vi "SET_START_STOP_MEASURE.vi"(7 "LabVIEW Web Service Request":refnum<class "Web Request.lvclass">, 10 "TRIGGER":bool=TRUE, 11 "DEVICE_SN":string) -> (3 "Response":T1)   [LabVIEW 2015]
uses:
  <vilib>/wsapi/Web Request.lvclass
  Share Data/uPower_kit.ctl
panel:
  # "Use the Web Service Request input terminal to call the VIs on the Web Services palette. Do not remove it from the connector pane unless you don't need access to the palette."
  # "Each additional control wired to the connector pane will be available as an input in the URL. To include an indicator in terminal-mode output (the default setting), it must also be wired to the connector pane."
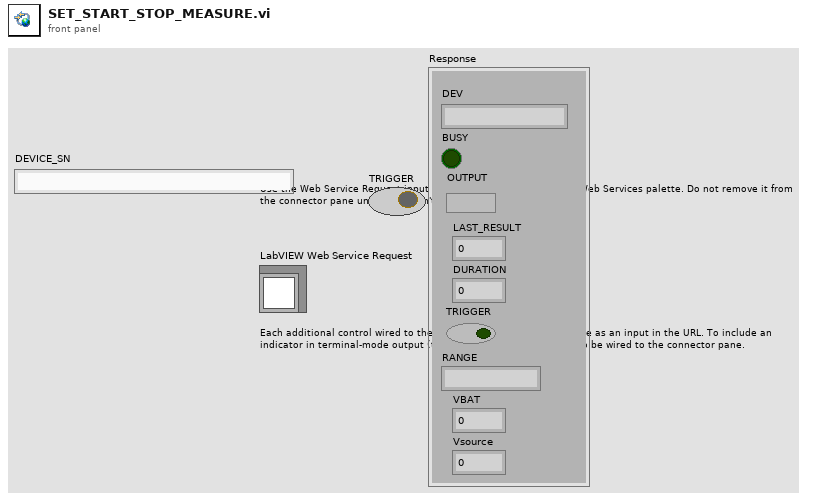
[diagram p1: front panel]
types:
  T1 = typedef "uPower_kit.ctl" = cluster{"DEV":string, "BUSY":bool, "VBAT":dbl, "OUTPUT":bool, "LAST_RESULT":dbl, "DURATION":u16, "TRIGGER":bool, "RANGE":string, "Vsource":dbl}
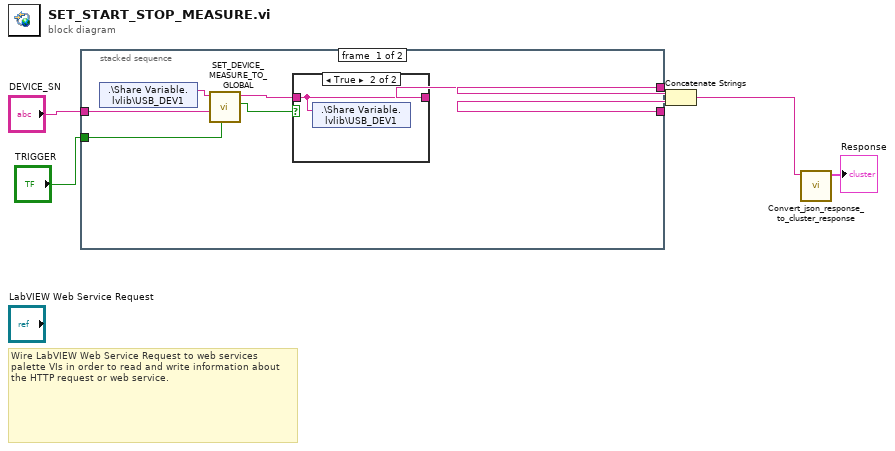
[diagram p0: block diagram]
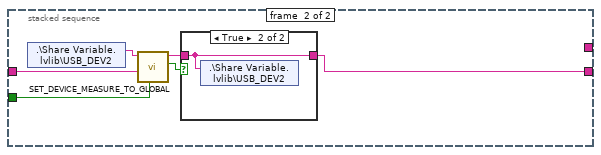
[diagram p3: hidden frame]
diagram:
  # "Wire LabVIEW Web Service Request to web services palette VIs in order to read and write information about the HTTP request or web service."
  n1 = stacked-sequence {
    tunnel: "DEVICE_SN" -> [w11 w18]
    tunnel: "TRIGGER" -> [w10 w17]
    tunnel: [w7 _] -> w4
    tunnel: [_ w14] -> w3
    frame #0 {
      n2 = shared-variable ".\\Share Variable.lvlib\\USB_DEV1"() -> (w12:string)  [unwired: 1 in, 1 out]
      n3 = call "SET_DEVICE_MEASURE_TO_GLOBAL.vi"("TRIGGER"=w10, "DEVICE in"=w11, "USB_DEV"=w12) -> ("DEVICE? 2"=w9:bool, "JSON string response 2"=w8:string)  [unwired: 7 in]
      n4 = case shown="True" w9 {
        tunnel: w8 -> [_ w13]
        tunnel: [_ w13] -> w7
        frame False {
        }
        frame True {
          n5 = shared-variable ".\\Share Variable.lvlib\\USB_DEV1"(w13) -> ()  [unwired: 1 in, 1 out]
        }
      }
    }
    frame #1 {
      n6 = shared-variable ".\\Share Variable.lvlib\\USB_DEV2"() -> (w19:string)  [unwired: 1 in, 1 out]
      n7 = call "SET_DEVICE_MEASURE_TO_GLOBAL.vi"("TRIGGER"=w17, "DEVICE in"=w18, "USB_DEV"=w19) -> ("DEVICE? 2"=w16:bool, "JSON string response 2"=w15:string)  [unwired: 7 in]
      n8 = case shown="True" w16 {
        tunnel: w15 -> [_ w20]
        tunnel: [_ w20] -> w14
        frame False {
        }
        frame True {
          n9 = shared-variable ".\\Share Variable.lvlib\\USB_DEV2"(w20) -> ()  [unwired: 1 in, 1 out]
        }
      }
    }
  }
  n10 = Concatenate Strings(w4, w3) -> (w2:string)
  n11 = call "Convert_json_response_to_cluster_response.vi"("Json_Response_in"=w2) -> ("Response"=→"Response":T1)  [unwired: 10 in]
